vi "Inst.TSL210.GetPrivateEvents.vi"(8 "error in (no error)":errorcluster, 11 "Inst.TSL210 in":refnum<class "Inst.TSL210.lvclass">) -> (0 "error out":errorcluster, 2 "Inst.TSL210 Private Events":cluster{"MessageToProcess":refnum<user-event>}, 3 "Inst.TSL210 out":refnum<class "Inst.TSL210.lvclass">)   [LabVIEW 2019, in "Inst.TSL210.lvclass"]
uses:
  Inst.TSL210.lvclass
  Typedefs/PrivateEvents--Inst.TSL210.MessageToProcess.ctl
  <userlib>/LevyLab/Instrument Framework/SMOs/RemoteControl/Typedefs/Message--Cluster.ctl
  Inst.TSL210.lvclass/Inst.TSL210.ctl
  <userlib>/LevyLab/Instrument Framework/SMOs/RemoteControl/RemoteControl.lvclass
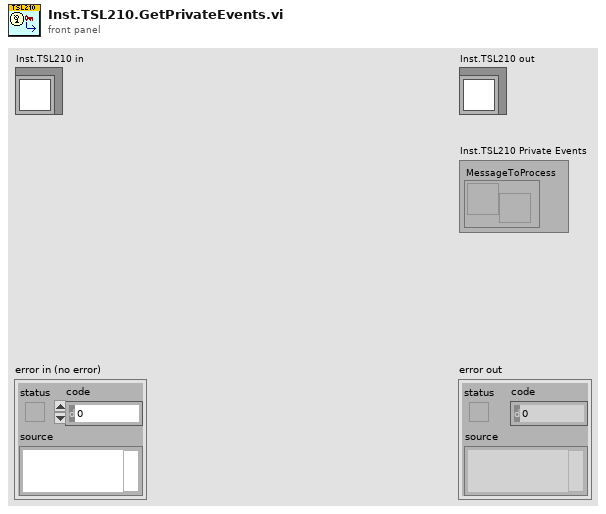
[diagram p1: front panel]
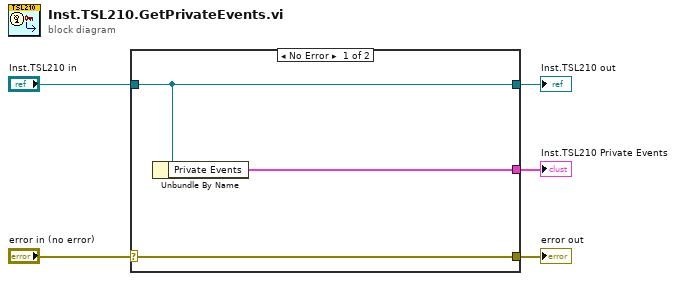
[diagram p0: block diagram]
diagram:
  n1 = case shown="No Error" "error in (no error)" {
    selector: "error in (no error)" -> [w8 w9]
    tunnel: [w8 w9] -> w4
    tunnel: [w7 w10] -> w2
    tunnel: "Inst.TSL210 in" -> [w7 w10]
    tunnel: [w6 _] -> w1
    frame No Error {
      n2 = Unbundle By Name(w7) -> ("Private Events"=w6:cluster{"MessageToProcess":refnum<user-event>})
    }
    frame Error {
    }
  }
  "error out" <- w4
  "Inst.TSL210 out" <- w2
  "Inst.TSL210 Private Events" <- w1
